vi "Create Test Method.vi"(8 "error in":errorcluster, 10 "Replacement VI":path=path "C:/Documents and Settings/Administrator/Desktop/Plugin Development/VI Tester Plugin/MyTestCase/testExample.vit", 11 "template test VI":path=path "C:/Documents and Settings/Administrator/Desktop/Plugin Development/VI Tester Plugin/MyTestCase/testExample.vit") -> (0 "error out":errorcluster, 2 "New VI Refnum":refnum<vi>)   [LabVIEW 2009]
uses:
  <vilib>/Utility/traverseref.llb/TRef TravTarget.ctl
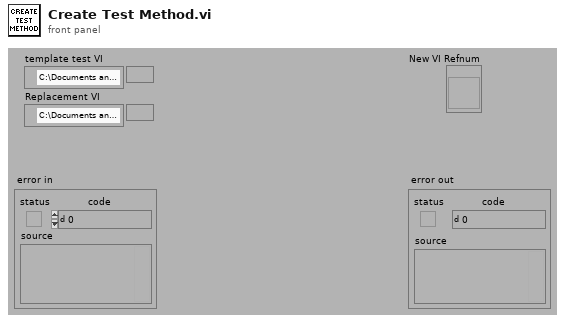
[diagram p1: front panel]
types:
  T1 = typedef "TRef TravTarget.ctl" = enum16{"FP", "BD", "Other"}
  T2 = enum32{"invalid VI type", "Standard VI", "Control VI", "Global VI", "Polymorphic VI", "Configuration VI", "SubSystem", "Facade VI", "Method VI", "Statechart Diagram VI"}
  T3 = enum16{"Invalid Wire Rule", "Required", "Recommended", "Optional", "Dynamic Dispatch"}[]
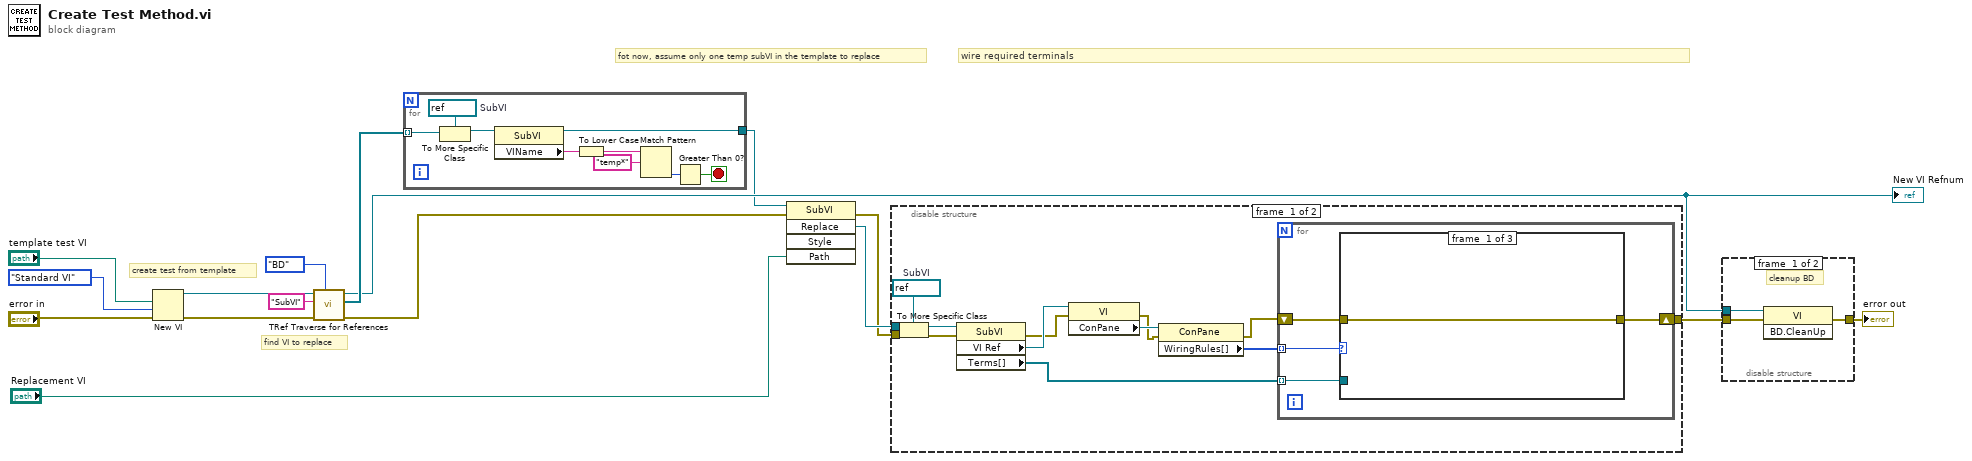
[diagram p0: block diagram]
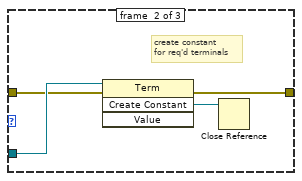
[diagram p2: hidden frame]
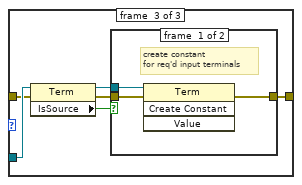
[diagram p3: hidden frame]
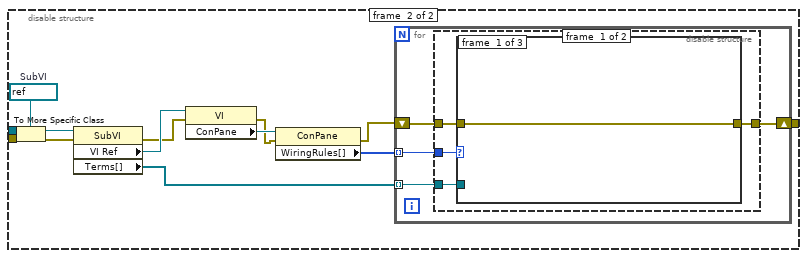
[diagram p5: hidden frame]
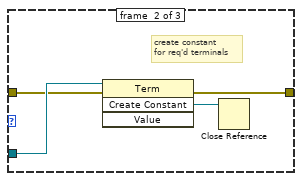
[diagram p6: hidden frame]
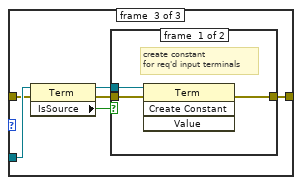
[diagram p7: hidden frame]
diagram:
  # "fot now, assume only one temp subVI in the template to replace"
  # "wire required terminals"
  # "find VI to replace"
  # "create test from template"
  n1 = New VI(8:"error in", 9:T2."Standard VI" ("vi type (standard vi)"), 10:"template test VI") -> (0:w12:errorcluster, 3:w15:refnum<vi>)  [unwired: 4 in]
  n2 = call <vilib>:"TRef Traverse for References.vi"("Traverse Target"=TRef_TravTarget."BD", "error in (no error)"=w12, "Class Name"="SubVI", "VI Refnum"=w15) -> ("error out"=w10:errorcluster, "References"=w14:refnum<vi>[], "dup VI Refnum"=w8:refnum<vi>)  [unwired: 4 in, 1 out]
  "New VI Refnum" <- w8
  n3 = for {
    tunnel: w14 -> [w25] mode=indexing
    tunnel: [w17] -> w5
    stop <- w18 stop-if-true
    w24 = refnum<vi> refnum  # SubVI
    n4 = To More Specific Class(target class=w24, reference=w25) -> (specific class reference=w23:refnum<vi>)  [unwired: 1 in, 1 out]
    n5 = property class="SubVI"(reference=w23) -> (reference out=w17:refnum<vi>, "VIName"=w22:string)  [unwired: 1 in, 1 out]
    n6 = To Lower Case(string=w22) -> (all lower case string=w20:string)
    n7 = Match Pattern(string=w20, regular expression="temp*") -> (offset past match=w19:i32)  [unwired: 1 in, 3 out]
    n8 = Greater Than 0?(x=w19) -> (x > 0?=w18:bool)
  }
  n9 = invoke class="SubVI" method="Replace"(reference=w5, error in=w10, "Path"="Replacement VI") -> (error out=w2:errorcluster, "Replace"=w3:refnum<vi>)  [unwired: 2 in, 3 out]
  n10 = disable-structure shown="Enabled" {
    disable-tunnel: [w29 w61] -> w6
    disable-tunnel: w3 -> [w27 w59]
    disable-tunnel: w2 -> [w26 w58]
    frame #0 {
      w28 = refnum<vi> refnum  # SubVI
      n11 = To More Specific Class(target class=w28, reference=w27, error in=w26) -> (specific class reference=w38:refnum<vi>, error out=w37:errorcluster)
      n12 = property class="SubVI"(reference=w38, error in=w37) -> (error out=w32:errorcluster, "VI Ref"=w36:refnum<vi>, "Terms[]"=w33:refnum<vi>[])  [unwired: 1 out]
      n13 = property class="VI"(reference=w36, error in=w32) -> (error out=w31:errorcluster, "ConPane"=w35:refnum<vi>)  [unwired: 1 out]
      n14 = property class="ConPane"(reference=w35, error in=w31) -> (error out=w30:errorcluster, "WiringRules[]"=w34:T3)  [unwired: 1 out]
      n15 = for {
        tunnel: w34 -> [w42] mode=indexing
        tunnel: w33 -> [w41] mode=indexing
        shift-right: [w39] -> w29
        shift-left: w30 -> [w40]
        n16 = case shown="\"Required\"" w42 {
          tunnel: w41 -> [_ w47 w52]
          tunnel: w40 -> [w43 w46 w50]
          tunnel: [w43 w45 w53] -> w39
          frame #0 {
          }
          frame #1 {
            # "create constant\nfor req'd terminals"
            n17 = invoke class="Term" method="Create Constant"(reference=w47, error in=w46) -> (error out=w45:errorcluster, "Create Constant"=w44:refnum<vi>)  [unwired: 2 in, 2 out]
            n18 = Close Reference(reference=w44) -> ()  [unwired: 1 in, 1 out]
          }
          frame #2 {
            n19 = property class="Term"(reference=w52, error in=w50) -> (reference out=w51:refnum<vi>, error out=w49:errorcluster, "IsSource"=w48:bool)
            n20 = case shown="False" w48 {
              tunnel: [w56 w57] -> w53
              tunnel: w51 -> [w55 _]
              tunnel: w49 -> [w54 w57]
              frame #0 {
                # "create constant\nfor req'd input terminals"
                n21 = invoke class="Term" method="Create Constant"(reference=w55, error in=w54) -> (error out=w56:errorcluster)  [unwired: 2 in, 3 out]
              }
              frame #1 {
              }
            }
          }
        }
      }
    }
    frame #1 {
      w60 = refnum<vi> refnum  # SubVI
      n22 = To More Specific Class(target class=w60, reference=w59, error in=w58) -> (specific class reference=w70:refnum<vi>, error out=w69:errorcluster)
      n23 = property class="SubVI"(reference=w70, error in=w69) -> (error out=w64:errorcluster, "VI Ref"=w68:refnum<vi>, "Terms[]"=w65:refnum<vi>[])  [unwired: 1 out]
      n24 = property class="VI"(reference=w68, error in=w64) -> (error out=w63:errorcluster, "ConPane"=w67:refnum<vi>)  [unwired: 1 out]
      n25 = property class="ConPane"(reference=w67, error in=w63) -> (error out=w62:errorcluster, "WiringRules[]"=w66:T3)  [unwired: 1 out]
      n26 = for {
        tunnel: w66 -> [w74] mode=indexing
        tunnel: w65 -> [w73] mode=indexing
        shift-right: [w71] -> w61
        shift-left: w62 -> [w72]
        n27 = disable-structure shown="Enabled" {
          disable-tunnel: w74 -> [w78 _]
          disable-tunnel: w73 -> [w77 _]
          disable-tunnel: w72 -> [w76 w94]
          disable-tunnel: [w75 w94] -> w71
          frame #0 {
            n28 = case shown="\"Dynamic Dispatch\"" w78 {
              tunnel: w77 -> [_ w83 w88]
              tunnel: w76 -> [w79 w82 w86]
              tunnel: [w79 w81 w89] -> w75
              frame #0 {
              }
              frame #1 {
                # "create constant\nfor req'd terminals"
                n29 = invoke class="Term" method="Create Constant"(reference=w83, error in=w82) -> (error out=w81:errorcluster, "Create Constant"=w80:refnum<vi>)  [unwired: 2 in, 2 out]
                n30 = Close Reference(reference=w80) -> ()  [unwired: 1 in, 1 out]
              }
              frame #2 {
                n31 = property class="Term"(reference=w88, error in=w86) -> (reference out=w87:refnum<vi>, error out=w85:errorcluster, "IsSource"=w84:bool)
                n32 = case shown="False" w84 {
                  tunnel: [w92 w93] -> w89
                  tunnel: w87 -> [w91 _]
                  tunnel: w85 -> [w90 w93]
                  frame #0 {
                    # "create constant\nfor req'd input terminals"
                    n33 = invoke class="Term" method="Create Constant"(reference=w91, error in=w90) -> (error out=w92:errorcluster)  [unwired: 2 in, 3 out]
                  }
                  frame #1 {
                  }
                }
              }
            }
          }
          frame #1 {
          }
        }
      }
    }
  }
  n34 = disable-structure shown="Enabled" {
    disable-tunnel: w8 -> [w97 _]
    disable-tunnel: [w96 w98] -> w7
    disable-tunnel: w6 -> [w95 w98]
    frame #0 {
      # "cleanup BD"
      n35 = invoke class="VI" method="BD.CleanUp"(reference=w97, error in=w95) -> (error out=w96:errorcluster)  [unwired: 1 in, 2 out]
    }
    frame #1 {
    }
  }
  "error out" <- w7
